vi "Configure acquisition--VISA.vi"(8 "error in (no error)":errorcluster, 9 "Type":enum16{"On demand", "Continous"}(ring), 10 "Config parameters":T1 {"Probe Attenuation" items=["1"=1, "10"=10, "20"=20, "50"=50, "100"=100, "500"=500, "1000"=1000]; "Channel" items=["Channel 1", "Channel 2", "Channel 3", "Channel 4", "Math", "Reference A", "Reference B", "Reference C", "Reference D"]; "Averaged Waveforms" items=["4"=4, "16"=16, "64"=64, "128"=128]; "Acquisition Type" items=["Sample", "Average", "Peak Detect"]}, 11 "VISA Refnum in":refnum<visa-resource-name>) -> (0 "error out":errorcluster, 3 "VISA resource name out":refnum<visa-resource-name>)   [LabVIEW 2020, in "TDS1002 Oscilloscope.lvlib"]
uses:
  TDS1002 Oscilloscope.lvlib
  Support/Channel configuration--cluster.ctl
  <instrlib>/Tektronix TDS 200 1000 2000 Series/Tektronix TDS 200 1000 2000 Series.lvlib
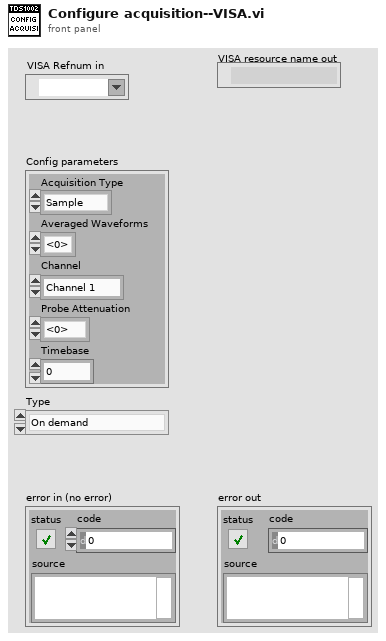
[diagram p1: front panel]
types:
  T1 = typedef "TDS1002 Oscilloscope.lvlib/Channel configuration--cluster.ctl" = cluster{"Acquisition Type":i32, "Averaged Waveforms":i32, "Channel":i32, "Probe Attenuation":i32, "Timebase":dbl}
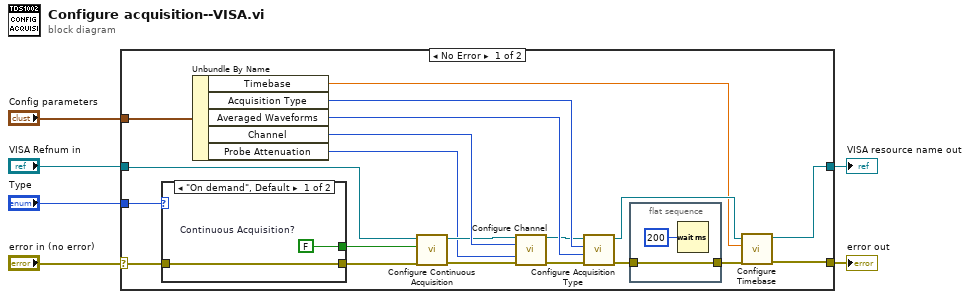
[diagram p0: block diagram]
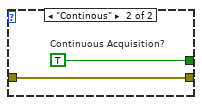
[diagram p2: hidden frame]
diagram:
  n1 = case shown="No Error" "error in (no error)" {
    selector: "error in (no error)" -> [w15 w33]
    tunnel: "Config parameters" -> [w23 _]
    tunnel: [w13 w33] -> w5
    tunnel: "VISA Refnum in" -> [w18 w34]
    tunnel: "Type" -> [w14 _]
    tunnel: [w11 w34] -> w1
    frame No Error {
      n2 = case shown="\"On demand\", Default" w14 {
        tunnel: w15 -> [w30 w32]
        tunnel: [w30 w32] -> w16
        tunnel: [w29 w31] -> w17
        frame "On demand", Default {
          w29 = FALSE  # Continuous Acquisition?
        }
        frame "Continous" {
          w31 = TRUE  # Continuous Acquisition?
        }
      }
      n3 = Unbundle By Name(w23) -> ("Timebase"=w10:dbl, "Acquisition Type"=w24:i32, "Averaged Waveforms"=w25:i32, "Channel"=w26:i32, "Probe Attenuation"=w9:i32)
      n4 = call <instrlib>:"Configure Continuous Acquisition.vi"("error in (no error)"=w16, "Enable Continuous Acquisition Mode (True)"=w17, "VISA resource name"=w18) -> ("error out"=w19:errorcluster, "VISA resource name out"=w20:refnum<visa-resource-name>)  [unwired: 7 out]
      n5 = call <instrlib>:"Configure Channel.vi"("VISA resource name"=w20, "Channel (0: Channel 1)"=w26, "Probe Attenuation (10: 10X)"=w9, "error in (no error)"=w19) -> ("VISA resource name out"=w22:refnum<visa-resource-name>, "error out"=w21:errorcluster)  [unwired: 10 in]
      n6 = call <instrlib>:"Configure Acquisition Type.vi"("error in (no error)"=w21, "Number of Averaged Waveforms (4: 4)"=w25, "Acquisition Type (0: Sample)"=w24, "VISA resource name"=w22) -> ("error out"=w8:errorcluster, "VISA resource name out"=w12:refnum<visa-resource-name>)  [unwired: 6 in]
      n7 = flat-sequence {
        tunnel: w8 -> [w28]
        tunnel: [w28] -> w7
        frame #0 {
          n8 = Wait (ms)(milliseconds to wait=u32 200) -> ()  [unwired: 1 out]
        }
      }
      n9 = call <instrlib>:"Configure Timebase.vi"("error in (no error)"=w7, "Timebase (0.0005 s)"=w10, "VISA resource name"=w12) -> ("error out"=w13:errorcluster, "VISA resource name out"=w11:refnum<visa-resource-name>)  [unwired: 7 in]
    }
    frame Error {
    }
  }
  "error out" <- w5
  "VISA resource name out" <- w1
